vi "DrawChessboardSpotOnSquare.vi"(0 "Bounds":T1, 1 "Black On White":bool, 4 "picture in":picture) -> (7 "picture out":picture)   [LabVIEW 2020, in "g_ar_toolkit.feature_detection.lvlib"]
uses:
  g_ar_toolkit.feature_detection.lvlib
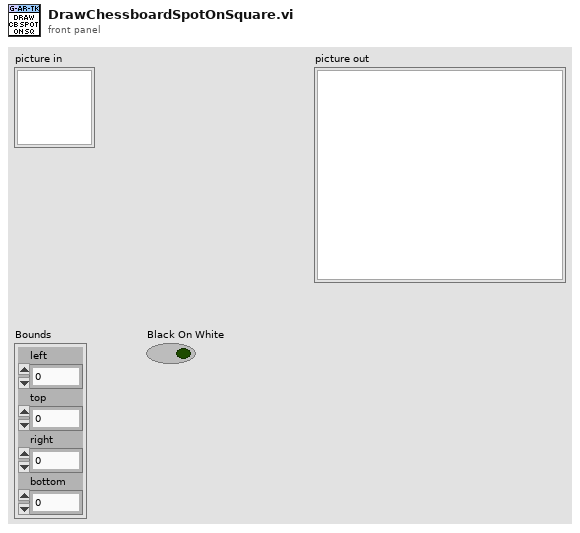
[diagram p1: front panel]
types:
  T1 = cluster{"left":i16, "top":i16, "right":i16, "bottom":i16}
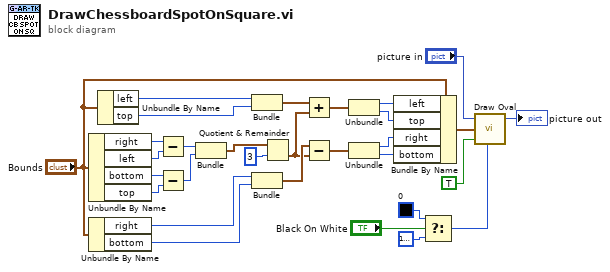
[diagram p0: block diagram]
diagram:
  n1 = Unbundle By Name("Bounds") -> ("right"=w28:i16, "left"=w27:i16, "bottom"=w26:i16, "top"=w25:i16)
  n2 = Unbundle By Name("Bounds") -> ("right"=w12:i16, "bottom"=w11:i16)
  n3 = Unbundle By Name("Bounds") -> ("left"=w14:i16, "top"=w15:i16)
  n4 = Subtract(x=w28, y=w27) -> (x-y=w24:i16)
  n5 = Subtract(x=w26, y=w25) -> (x-y=w23:i16)
  n6 = Bundle(w24, w23) -> (w22:cluster{i16, i16})  [unwired: 1 in]
  n7 = Bundle("left"=w14, "top"=w15) -> (w13:cluster{"left":i16, "top":i16})  [unwired: 1 in]
  n8 = Bundle("right"=w12, "bottom"=w11) -> (w10:cluster{"right":i16, "bottom":i16})  [unwired: 1 in]
  n9 = Quotient & Remainder(x=w22, y=i16 3) -> (floor(x/y)=w9:cluster{i16, i16})  [unwired: 1 out]
  n10 = Add(x=w13, y=w9) -> (x+y=w7:cluster{i16, i16})
  n11 = Subtract(x=w10, y=w9) -> (x-y=w4:cluster{i16, i16})
  n12 = Unbundle(w7) -> (w6:i16, w5:i16)
  n13 = Unbundle(w4) -> (w3:i16, w2:i16)
  n14 = Bundle By Name(cluster="Bounds", "left"=w6, "top"=w5, "right"=w3, "bottom"=w2) -> (w1:T1)
  n15 = Select(t=u32 0 ("color(black)"), s="Black On White", f=u32 16777225 ("color(black)")) -> (s? t:f=w18:u32)
  n16 = call <vilib>:"Draw Oval.vi"("picture"="picture in", "rect"=w1, "fill?(F)"=TRUE, "color(black)"=w18) -> ("new picture"=→"picture out":picture)  [unwired: 5 in]
